vi "Register Logger.vi"(8 "error in (no error)":errorcluster, 9 "Task ID":string, 10 "EnQr":refnum<class "Message Enqueuer.lvclass">, 11 "LoggingManager in":refnum<class "LoggingManager.lvclass">) -> (0 "error out":errorcluster, 3 "LoggingManager out":refnum<class "LoggingManager.lvclass">)   [LabVIEW 2020, in "Volatus.lvlib" / "LoggingManager.lvclass"]
uses:
  LoggingManager.lvclass
  C:/dev/lv20CE/relink/lv-volatus/Volatus/Task/Task.lvclass
  <vilib>/ActorFramework/Message Enqueuer/Message Enqueuer.lvclass
  LoggingManager.lvclass/LoggingManager.ctl
  Task/Task.lvclass/Task.ctl
  VolatusAPI/VolatusAPI.lvclass/VolatusAPI.ctl
  Event API/EventAPI.lvclass/EventAPI.ctl
  EventHandler Messages/Handle Event Msg/Handle Event Msg.lvclass/Handle Event Msg.ctl
  <vilib>/ActorFramework/Message Enqueuer/Message Enqueuer.lvclass/Message Enqueuer.ctl
  EventHandler Messages/Handle Event Msg/Send Handle Event.vi
  <vilib>/ActorFramework/Message Enqueuer/Enqueue.vi
  EventHandler Messages/Handle Event Msg/Handle Event Msg.lvclass
  C:/Program Files (x86)/National Instruments/LabVIEW 2020/vi.lib/ActorFramework/Message/Message.lvclass
  <vilib>/ActorFramework/Message Priority Queue/Priority Enqueue.vi
  Task/Task.lvclass
  LoggingHandler Messages/Set Logging Root Msg/Set Logging Root Msg.lvclass
  C:/Program Files (x86)/National Instruments/LabVIEW 2020/vi.lib/ActorFramework/Actor/Actor.lvclass
  C:/dev/lv20CE/relink/lv-volatus/Volatus/TaskStateHandler/TaskStateHandler.lvclass
  C:/dev/lv20CE/relink/lv-volatus/Volatus/VectoMessageHandler/VectoMessageHandler.lvclass
  C:/dev/lv20CE/relink/lv-volatus/Volatus/LoggingManager/LoggingManager.lvclass
  C:/dev/lv20CE/relink/lv-volatus/Volatus/API Provider/API Provider.lvclass
  C:/dev/lv20CE/relink/lv-volatus/Volatus/LoggingHandler/LoggingHandler.lvclass
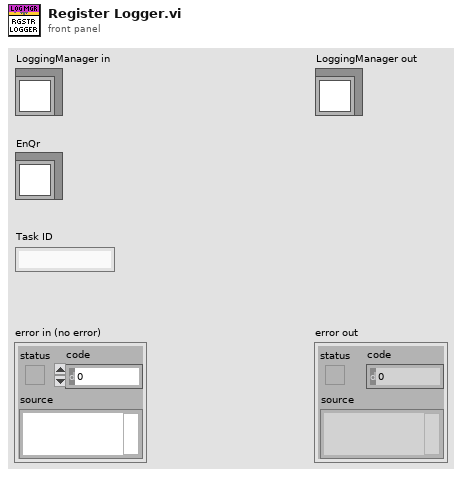
[diagram p1: front panel]
types:
  T1 = map{string, refnum<class "Message Enqueuer.lvclass">}
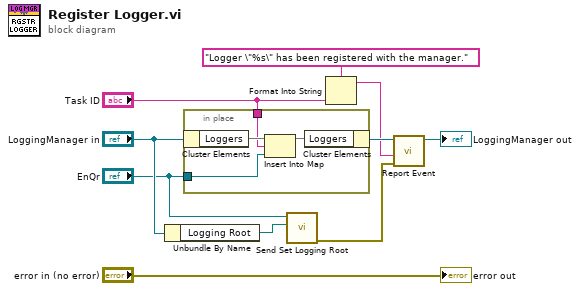
[diagram p0: block diagram]
diagram:
  n1 = Unbundle By Name("LoggingManager in") -> ("Logging Root"=w3:path)
  n2 = in-place {
    in-place-border: "Task ID" -> [w13]
    in-place-border: "EnQr" -> [w12]
    n3 = in-place-cluster #1("LoggingManager in") -> ("Loggers"=w14:T1)
    n4 = Insert Into Map(map in=w14, key=w13, value=w12) -> (map out=w11:T1)  [unwired: 2 out]
    n5 = in-place-cluster #1("Loggers"=w11) -> (w9:refnum<class "LoggingManager.lvclass">)
  }
  n6 = call "Send Set Logging Root.vi"("LoggingRoot"=w3, "Message Enqueuer"="EnQr") -> ("error out"=w1:errorcluster)  [unwired: 8 in, 1 out]
  n7 = Format Into String(format string="Logger \"%s\" has been registered with the manager.", "Task ID") -> (resulting string=w5:string)  [unwired: 2 in, 1 out]
  n8 = call "Report Event.vi"("error in (no error)"=w1, "Message"=w5, "Task in"=w9) -> ("Task out"=→"LoggingManager out":refnum<class "LoggingManager.lvclass">)  [unwired: 7 in, 1 out]
  "error out" <- "error in (no error)"
